vi "lockin - replace AO DC.vi"(8 "error in (no error)":errorcluster, 10 "AO.DC (V)":dbl[](array[numeric]), 11 "LockinDAQ":refnum<class "Lockin.DAQ.lvclass">=refnum) -> (0 "error out":errorcluster, 3 "LockinDAQ out":refnum<class "Lockin.DAQ.lvclass">)   [LabVIEW 2016, in "Lockin.DAQ.lvclass"]
uses:
  Lockin.DAQ.lvclass
  Lockin.DAQ.lvclass/Lockin.DAQ.ctl
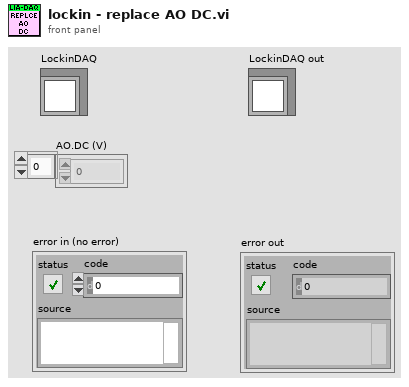
[diagram p1: front panel]
types:
  T1 = typedef "Lockin.DAQ.lvclass/AO-cluster.ctl" = cluster{"Ch":i32[], "Amp (V)":dbl[], "DC (V)":dbl[], "f (Hz)":dbl[], "Phase (°)":dbl[], "Function":T2[], "Sweep?":bool[]}
  T2 = typedef "Lockin.DAQ.lvclass/Function-enum.ctl" = enum16{"Sine", "Triangle", "Square", "Sawtooth"}
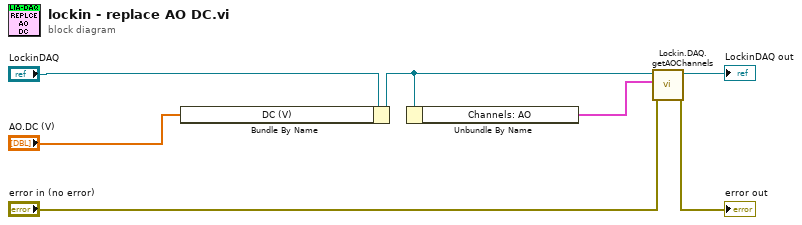
[diagram p0: block diagram]
diagram:
  n1 = Bundle By Name(cluster="LockinDAQ", "DC (V)"="AO.DC (V)") -> (w6:refnum<class "Lockin.DAQ.lvclass">)
  n2 = Unbundle By Name(w6) -> ("Channels: AO"=w1:T1)
  n3 = call "Lockin.DAQ.getAOChannels.vi"("error in (no error)"="error in (no error)", "Channels: AO"=w1, "LockinDAQ"=w6) -> ("error out"=→"error out":errorcluster, "LockinDAQ out"=→"LockinDAQ out":refnum<class "Lockin.DAQ.lvclass">)  [unwired: 7 in]
